vi "Write String Array to Spreadsheet With Header.vi"(0 "file path (dialog if empty)":path, 1 "Header":string, 5 "delimiter (\\t)":string="\t", 7 "Data String Array":string[][](array[string]), 9 "append to file? (new file:F)":bool, 11 "error in (no error)":errorcluster, 12 "transpose? (no:F)":bool) -> (4 "new file path (Not A Path if cancelled)":path, 15 "error out":errorcluster)   [LabVIEW 2017]
doc: "Converts a 2D or 1D array of strings, signed integers, or double-precision numbers to a text string and writes the string to a new byte stream file or appends the string to an existing file. Wire data to the <B>2D data</B> input or <B>1D data</B> input to determine the polymorphic instance to use or manually select the instance.\n\nUse this VI to transpose or separate data.\n\n<B>Note</B> To format with Microsoft Excel, use ActiveX with LabVIEW or the Report Generation Toolkit for Microsoft Office."
panel:
  in  "prompt":string="Choose file to write."
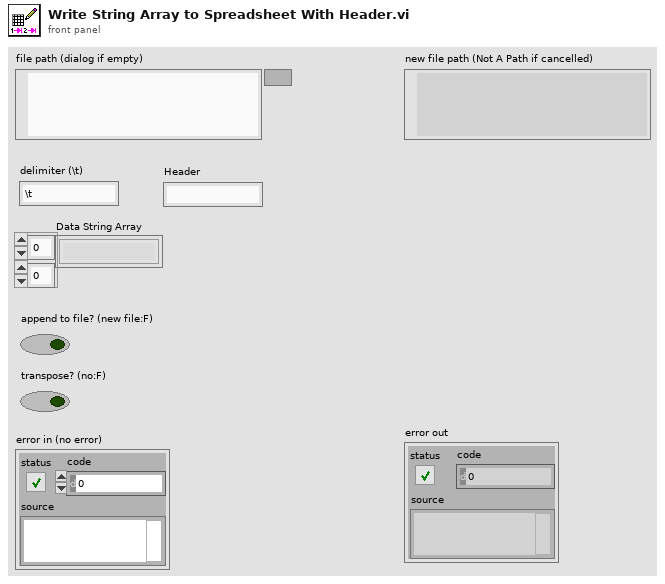
[diagram p1: front panel]
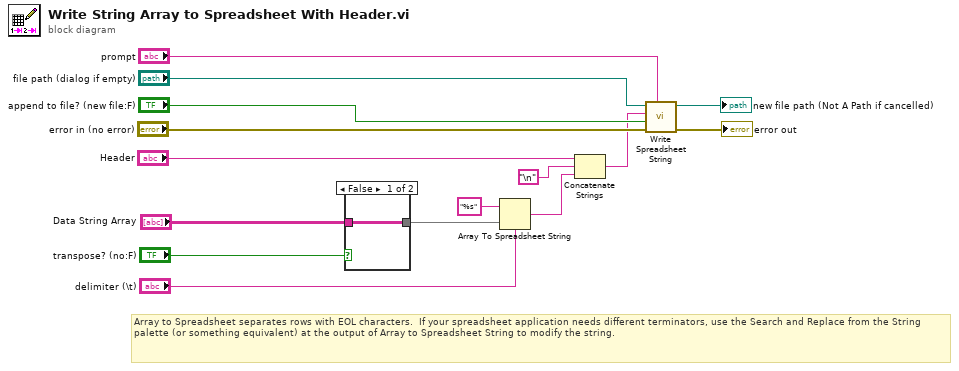
[diagram p0: block diagram]
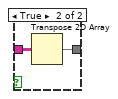
[diagram p2: hidden frame]
diagram:
  # "Array to Spreadsheet separates rows with EOL characters.  If your spreadsheet application needs different terminators, use the Search and Replace from the String palette (or something equivalent) at the output of Array to Spreadsheet String to modify the string."
  n1 = case shown="False" "transpose? (no:F)" {
    tunnel: [w16 w18] -> w13
    tunnel: "Data String Array" -> [w16 w17]
    frame False {
    }
    frame True {
      n2 = Transpose 2D Array(2D array=w17) -> (transposed array=w18:string[][])
    }
  }
  n3 = Array To Spreadsheet String(delimiter (Tab)="delimiter (\\t)", array=w13, 3:"%s" ("format string")) -> (spreadsheet string=w4:string)
  n4 = Concatenate Strings("Header", "\n", w4) -> (w3:string)
  n5 = call <vilib>:"Write Spreadsheet String.vi"("prompt"="prompt", "error in"="error in (no error)", "append to file? (new file:F)"="append to file? (new file:F)", "spreadsheet string"=w3, "file path (dialog if empty)"="file path (dialog if empty)") -> ("error out"=→"error out":errorcluster, "path"=→"new file path (Not A Path if cancelled)":path)  [unwired: 5 in]
